vi "Create Flattened FIFO Header.vi"(8 "error in (no error)":errorcluster, 9 "Payload Length":i32, 10 "FIFO Timestamps":T1, 11 "CIFChannels in":refnum<class "CIFChannels.lvclass">) -> (0 "error out":errorcluster, 2 "Flattened FIFO Header":u8[](array[numeric]) format="%.0x", 3 "CIFChannels out":refnum<class "CIFChannels.lvclass">)   [LabVIEW 2021, in "CIFChannels.lvclass"]
uses:
  CIFChannels.lvclass
  ChannelCommon/typedef/TimeStamps.ctl
  CIFChannels.lvclass/CIFChannels.ctl
  <vilib>/CIF Foundation/CIF Utilities/DataTypes/Flatten Unflatten/Flatten U64.vi
  <vilib>/CIF Foundation/CIF Utilities/DataTypes/Flatten Unflatten/Flatten I64.vi
  <vilib>/CIF Foundation/CIF Utilities/Time/System Time/Get System Time.vi
  <vilib>/CIF Foundation/CIF Utilities/Time/System Time/LabVIEW Time to TAI Time.vi
  ChannelCommon/ChannelCommon.lvlib
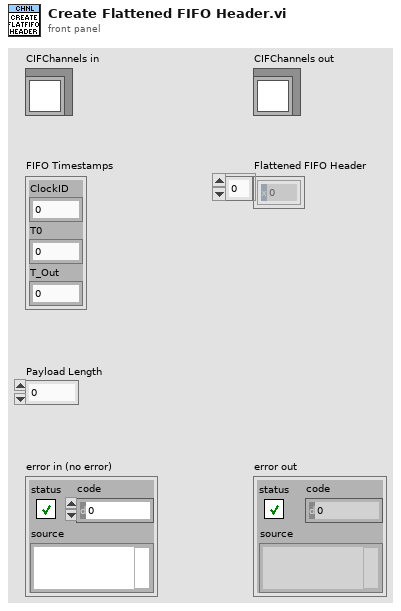
[diagram p1: front panel]
types:
  T1 = typedef "ChannelCommon.lvlib/TimeStamps.ctl" = cluster{"ClockID":u8, "T0":i64, "T_Out":i64}
  T2 = typedef "ChannelCommon.lvlib/FIFO Header.ctl" = cluster{"Length":u64, "T0":i64, "T_Out":i64, "T_Tx":i64, "Ctr":u64, "ClockID":u8}
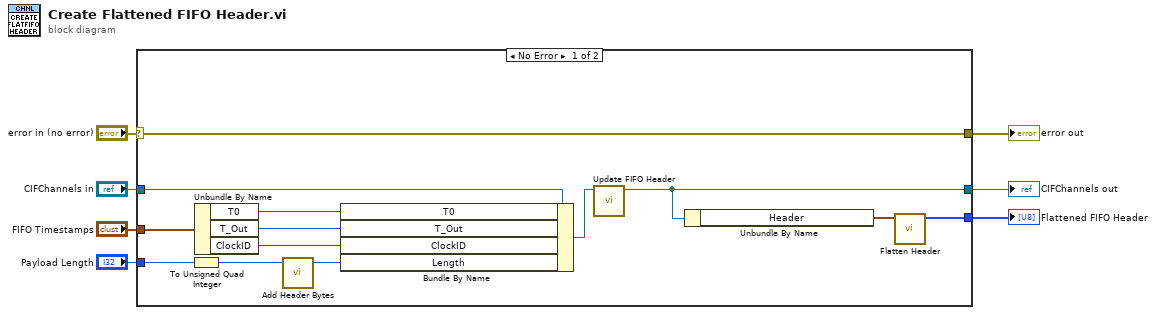
[diagram p0: block diagram]
diagram:
  n1 = case shown="No Error" "error in (no error)" {
    selector: "error in (no error)" -> [w10 w22]
    tunnel: [w10 w22] -> w4
    tunnel: [w14 w21] -> w3
    tunnel: "CIFChannels in" -> [w12 w21]
    tunnel: "FIFO Timestamps" -> [w20 _]
    tunnel: [w13 _] -> w2
    tunnel: "Payload Length" -> [w11 _]
    frame No Error {
      n2 = To Unsigned Quad Integer(1:w11) -> (0:w9:u64)
      n3 = Unbundle By Name(w20) -> ("T0"=w19:i64, "T_Out"=w18:i64, "ClockID"=w17:u8)
      n4 = call "Add Header Bytes.vi"("Bytes/Msg"=w9) -> ("Bytes/Msg with header"=w8:u64)  [unwired: 3 in]
      n5 = Bundle By Name(cluster=w12, "T0"=w19, "T_Out"=w18, "ClockID"=w17, "Length"=w8) -> (w16:refnum<class "CIFChannels.lvclass">)
      n6 = call "Update FIFO Header.vi"("CIFChannels in"=w16) -> ("CIFChannels out"=w14:refnum<class "CIFChannels.lvclass">)  [unwired: 10 in]
      n7 = Unbundle By Name(w14) -> ("Header"=w15:T2)
      n8 = call "Flatten Header.vi"("Header in"=w15) -> ("Flattened Data out"=w13:u8[])  [unwired: 10 in]
    }
    frame Error {
    }
  }
  "error out" <- w4
  "CIFChannels out" <- w3
  "Flattened FIFO Header" <- w2
